vi "DateTimeString Manipulation.vi"(5 "FPU DT String":string) -> (2 "FPF DT String":string)   [LabVIEW 2014]
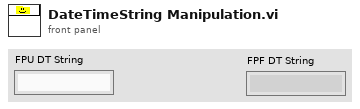
[diagram p1: front panel]
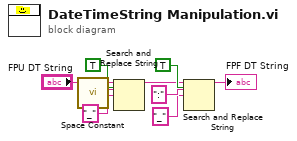
[diagram p0: block diagram]
diagram:
  n1 = call <vilib>:"Space Constant.vi"() -> ("String"=w8:string)
  n2 = Search and Replace String(replace all?=TRUE ("replace all? (F)"), input string="FPU DT String", search string=w8, replace string="_") -> (result string=w2:string)  [unwired: 4 in, 3 out]
  n3 = Search and Replace String(replace all?=TRUE ("replace all? (F)"), input string=w2, search string=":", replace string="_") -> (result string=→"FPF DT String":string)  [unwired: 4 in, 3 out]
